vi "lab 5.vi"() -> ()   [LabVIEW 2010]
uses:
  <vilib>/Utility/file.llb/Write To Spreadsheet File (I64).vi
panel:
  in  "Data File Path Ending":string
  out "Date/Time String":string
  in  "Time Format String (%c)":string
  in  "Auto Save Data":bool
  out "Current Acquisition":u16[](graph)
  out "Previous Acquisition":u16[](graph)
  in  "Inner Channel Delay":sgl=-1.0
  in  "Range":i32(ring)=1 items=["Not Programmable"=0, "+- 20 V"=27, "+- 10 V"=1, "+- 5 V"=2, "+- 4 V"=28, "+- 2.5 V"=3, "+- 2 V"=29, "+- 1.67 V"=4, "+- 1.25 V"=5, "+- 1 V"=6, "+- .625 V"=7, "+- .5 V"=8, "+- .25 V"=30, "+- .2 V"=31, "+- .1 V"=9, "+- .05 V"=10, "+- .01 V"=11, "+- .005 V"=12, "0 - 10 V"=13, "0 - 5 V"=14, "0 - 4 V"=36, "0 - 2.5 V"=15, "0 - 2 V"=16, "0 - 1.67 V"=17, "0 - 1.25 V"=18, "0 - 1 V"=19, "0 - .5 V"=32, "0 - .25 V"=33, "0 - .2 V"=34, "0 - .1 V"=20, "0 - .02 V"=35, "0 - .01 V"=21, "4 - 20 mA"=22, "2 - 10 mA"=23, "1 - 5 mA"=24, ".5 - 2.5 mA"=25, "0 - 20 mA"=26]
  in  "Rate":i32=1000
  in  "Options":i32
  in  "Count":i32=1000
  in  "LowChan":i32
  in  "HighChan":i32
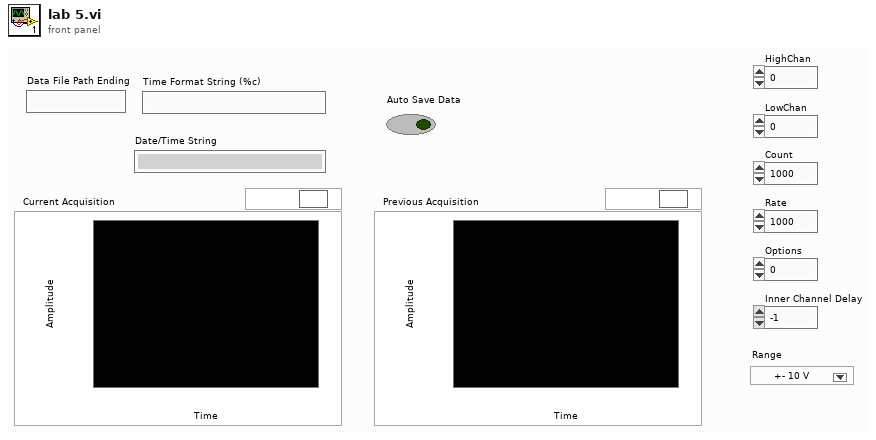
[diagram p1: front panel]
types:
  T1 = typedef "imagedata.ctl" = cluster{"image type":i32, "image depth":i32, "image":u8[], "mask":u8[], "colors":u32[], "Rectangle":cluster{"left":i16, "top":i16, "right":i16, "bottom":i16}}
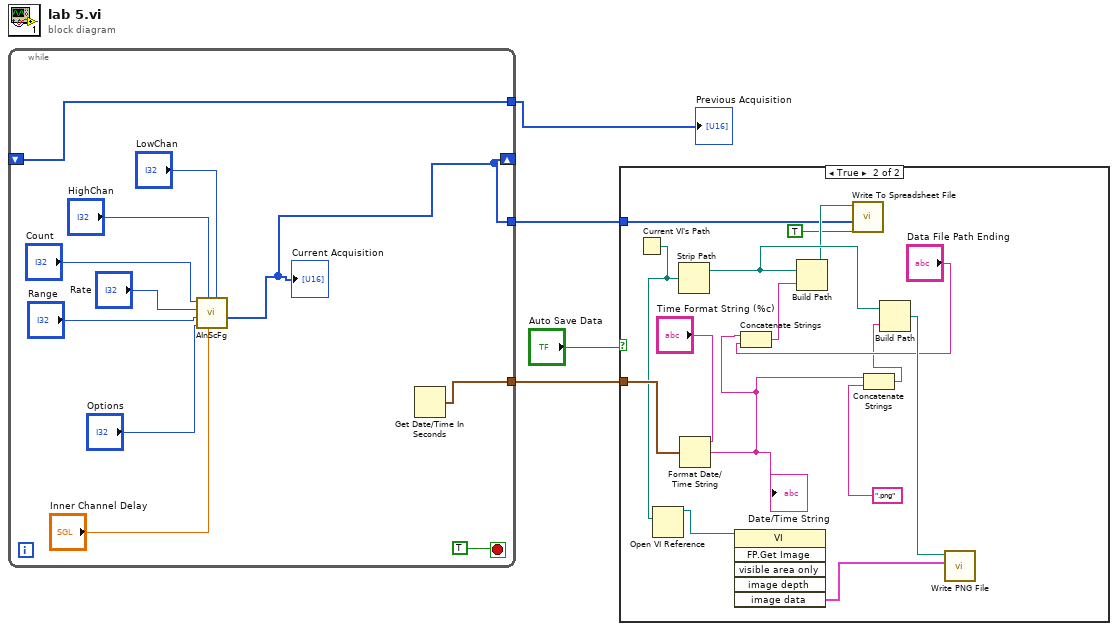
[diagram p0: block diagram]
diagram:
  n1 = while {
    shift-right: [w6] -> _
    shift-left: _ -> [w7]
    tunnel: [w7] -> w4
    tunnel: [w6] -> w2
    tunnel: [w5] -> w1
    stop <- TRUE stop-if-true
    n2 = call <menus>:"AInScFg.VI"("LowChan"="LowChan", "InterChannel Delay"="Inner Channel Delay", "HighChan"="HighChan", "Options"="Options", "Range"="Range", "Rate"="Rate", "Count"="Count") -> ("ADData"=w6:u16[])  [unwired: 1 in, 2 out]
    "Current Acquisition" <- w6
    n3 = Get Date/Time In Seconds() -> (seconds since 1Jan1904=w5:timestamp)
  }
  "Previous Acquisition" <- w4
  n4 = case shown="True" "Auto Save Data" {
    tunnel: w2 -> [_ w28]
    tunnel: w1 -> [_ w27]
    frame False {
    }
    frame True {
      n5 = Current VI's Path() -> (path=w26:path)
      n6 = Open VI Reference(vi path=w26) -> (vi reference=w23:refnum<vi>)  [unwired: 5 in, 1 out]
      n7 = Strip Path(path=w26) -> (stripped path=w30:path)  [unwired: 1 out]
      n8 = Format Date/Time String(time format string (%c)="Time Format String (%c)", seconds (now)=w27) -> (date/time string=w20:string)  [unwired: 1 in]
      "Date/Time String" <- w20
      n9 = invoke class="VI" method="FP.Get Image"(reference=w23) -> ("image data"=w25:T1)  [unwired: 5 in, 5 out]
      n10 = Concatenate Strings(w20, "Data File Path Ending") -> (w22:string)
      n11 = Build Path(base path=w30, name or relative path=w22) -> (appended path=w29:path)
      n12 = call-poly <vilib>:"Write To Spreadsheet File.vi"("append to file? (new file:F)"=TRUE, "1D data"=w28, "file path (dialog if empty)"=w29) -> ()  [unwired: 5 in, 1 out]
      n13 = Concatenate Strings(w20, ".png" ("string")) -> (w16:string)
      n14 = Build Path(base path=w30, name or relative path=w16) -> (appended path=w24:path)
      n15 = call <vilib>:"Write PNG File.vi"("image data"=w25, "path to PNG file"=w24) -> ()  [unwired: 8 in, 2 out]
    }
  }
